vi "Write TDM Channel Groups.vi"() -> ()   [LabVIEW 2023]
doc: "Writes channel groups to a TDM file."
uses:
  <vilib>/Platform/storage/lvStorage.llb/_openFunction.ctl
  <vilib>/Platform/storage/Storage.llb/usiSequenceRepresentation.ctl
  <vilib>/Platform/storage/Storage.llb/usiOverwriteOptions.ctl
  Instance           1 28Saved   Write Channel Groups .vi
  Instance           2 28Saved   Write Channel Groups .vi
  Instance           3 28Saved   Write Channel Groups .vi
  Instance           4 28Saved   Write Channel Groups .vi
  <vilib>/Platform/storage/lvStorage.llb/_openStorageWithRootAutoDetect.vi
  <vilib>/Platform/storage/lvStorage.llb/xStorage/xStorageSupp/ErrorOut.vi
  <vilib>/Platform/storage/Storage.llb/__savePropString.vi
  <vilib>/Platform/storage/Storage.llb/__savePropTime.vi
  <vilib>/Platform/storage/Storage.llb/_createExplicitChildObject.vi
  <vilib>/Platform/storage/lvStorage.llb/_prepDDT.vi
  <vilib>/Platform/storage/lvStorage.llb/_getChannelNameFromDDT.vi
  <vilib>/Platform/storage/lvStorage.llb/_createOrGetByNameExplicitChildObject.vi
  <vilib>/Platform/storage/lvStorage.llb/_saveDDT.vi
  <vilib>/Platform/storage/Storage.llb/Get Object Info.vi
  <vilib>/Platform/storage/Storage.llb/__closeStorageFromObject.vi
  <vilib>/Platform/storage/lvStorage.llb/xStorage/Open Data Storage/Open Data Storage.xnode
  <vilib>/Platform/storage/lvStorage.llb/xStorage/Set Properties/Set Properties.xnode
  <vilib>/Platform/storage/lvStorage.llb/xStorage/Write Data/Write Data.xnode
  <vilib>/Platform/storage/lvStorage.llb/xStorage/Close Data Storage/Close Data Storage.xnode
panel:
  out "Data Written to File (With Noise)":dynamicdata(graph)
  out "Data Written to File (No Noise)":dynamicdata(graph)
  # "Overview: Demonstrates the use of the DataPlugin Express VIs to write channel group data to a TDM file.\nRequirements: Windows\nInstructions:\n1. Run this VI.\n2. Open Read TDM Channel Groups.vi and follow the instructions on its front panel."
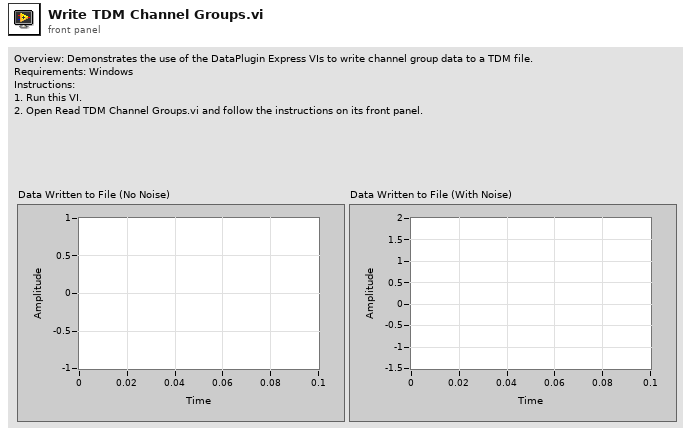
[diagram p1: front panel]
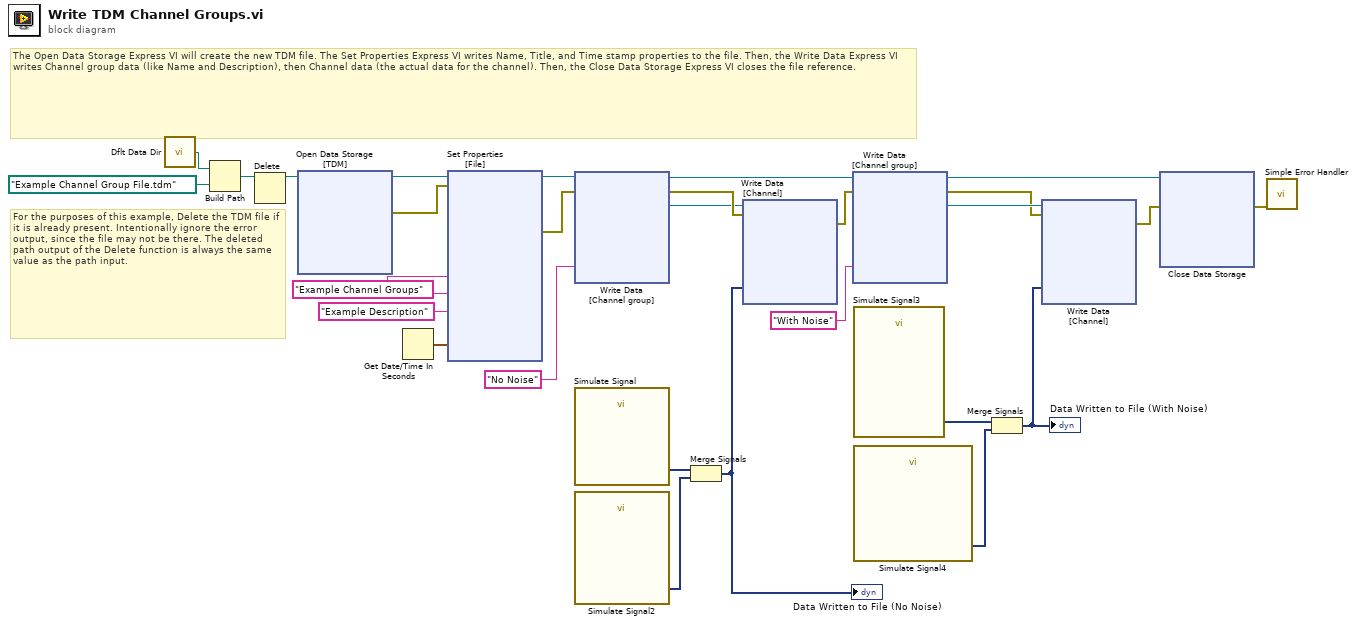
[diagram p0: block diagram]
diagram:
  w11 = "Example Description" ("title")
  w3 = "Example Channel Groups" ("name")
  # "The Open Data Storage Express VI will create the new TDM file. The Set Properties Express VI writes Name, Title, and Time stamp properties to the file. Then, the Write Data Express VI writes Channel group data (like Name and Description), then Channel data (the actual data for the channel). Then, the Close Data Storage Express VI closes the file reference."
  # "For the purposes of this example, Delete the TDM file if it is already present. Intentionally ignore the error output, since the file may not be there. The deleted path output of the Delete function is always the same value as the path input."
  n1 = call <vilib>:"Dflt Data Dir.vi"() -> ("App:Default Data Directory"=w5:path)
  n2 = Build Path(base path=w5, name or relative path=path "Example Channel Group File.tdm" ("default name")) -> (appended path=w7:path)
  n3 = Delete(path (use dialog)=w7) -> (deleted path=w4:path)  [unwired: 4 in, 2 out]
  n4 = xnode "Open Data Storage\n[TDM]"("file path"=w4) -> ("storage refnum (file)"=w9:refnum<k20>, "error out"=w14:errorcluster)  [unwired: 2 in, 3 out]
  n5 = Get Date/Time In Seconds() -> (seconds since 1Jan1904=w10:timestamp)
  n6 = xnode "Set Properties\n[File]"("Name"=w3, "Description"=w3, "Title"=w11, "Author"=w11, "Time stamp"=w10, "storage refnum (file)"=w9, "error in"=w14) -> ("storage refnum (file) out"=w13:refnum<k20>, "error out"=w12:errorcluster)
  n7 = xnode "Write Data\n[Channel group]"("Name"="No Noise" ("name"), "storage refnum (file)"=w13, "error in"=w12) -> ("storage refnum (file) out"=w22:refnum<k20>, "error out"=w27:errorcluster, "storage refnum (channel group)"=w26:refnum<k20>)
  n8 = call "Simulate Signal"() -> ("Sine"=w24:dynamicdata)  [unwired: 6 in, 9 out]
  n9 = call "Simulate Signal2"() -> ("Sawtooth"=w25:dynamicdata)  [unwired: 6 in, 9 out]
  n10 = Merge Signals(w24, w25) -> (w1:dynamicdata)
  "Data Written to File (No Noise)" <- w1
  n11 = xnode "Write Data\n[Channel]"("Signal"=w1, "storage refnum (channel group)"=w26, "error in"=w27) -> ("error out"=w21:errorcluster)  [unwired: 4 out]
  n12 = xnode "Write Data\n[Channel group]"("Name"="With Noise" ("name"), "storage refnum (file)"=w22, "error in"=w21) -> ("storage refnum (file) out"=w8:refnum<k20>, "error out"=w17:errorcluster, "storage refnum (channel group)"=w18:refnum<k20>)
  n13 = call "Simulate Signal3"() -> ("Sine with Noise"=w20:dynamicdata)  [unwired: 8 in, 7 out]
  n14 = call "Simulate Signal4"() -> ("Sawtooth with Noise"=w19:dynamicdata)  [unwired: 8 in, 7 out]
  n15 = Merge Signals(w20, w19) -> (w2:dynamicdata)
  "Data Written to File (With Noise)" <- w2
  n16 = xnode "Write Data\n[Channel]"("Signal"=w2, "storage refnum (channel group)"=w18, "error in"=w17) -> ("error out"=w16:errorcluster)  [unwired: 4 out]
  n17 = xnode "Close Data Storage\n"("storage refnum (file)"=w8, "error in (no error)"=w16) -> ("error out"=w15:errorcluster)  [unwired: 1 out]
  n18 = call <vilib>:"Simple Error Handler.vi"("error in (no error)"=w15) -> ()  [unwired: 1 in, 8 out]
